vi "permission group to mode_t.vi"(11 "permissions group":T1) -> (3 "mode_t":u32)   [LabVIEW 2016, in "Linux RT IPC.C.lvlib"]
uses:
  Linux RT IPC.C.lvlib
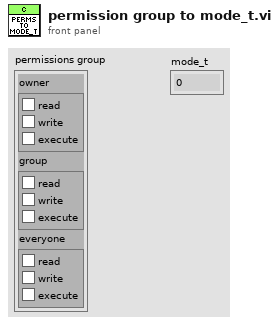
[diagram p1: front panel]
types:
  T1 = cluster{"owner":cluster{"read":bool, "write":bool, "execute":bool}, "group":cluster{"read":bool, "write":bool, "execute":bool}, "everyone":cluster{"read":bool, "write":bool, "execute":bool}}
  T2 = cluster{"read":bool, "write":bool, "execute":bool}
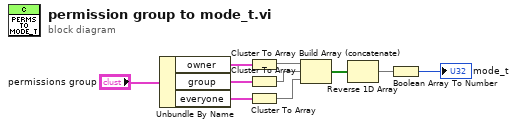
[diagram p0: block diagram]
diagram:
  n1 = Unbundle By Name("permissions group") -> ("owner"=w3:T2, "group"=w4:T2, "everyone"=w5:T2)
  n2 = Cluster To Array(cluster=w3) -> (array=w6:bool[])
  n3 = Cluster To Array(cluster=w4) -> (array=w7:bool[])
  n4 = Cluster To Array(cluster=w5) -> (array=w8:bool[])
  n5 = Build Array (concatenate)(w6, w7, w8) -> (w9:bool[])
  n6 = Reverse 1D Array(array=w9) -> (reversed array=w10:bool[])
  n7 = Boolean Array To Number(Boolean array=w10) -> (number=→"mode_t":u32)
